vi "Gain compensation.vi"(5 "A":dbl=1.2727, 7 "b":dbl=-0.169, 10 "sampling frequency":dbl=50.0, 11 "Data":dbl[](array[numeric])) -> (3 "compensated":dbl[](array[numeric]))   [LabVIEW 2012]
uses:
  <vilib>/Analysis/2dsp.llb/Real FFT.vi
  <vilib>/Analysis/2dsp.llb/Inverse Real FFT.vi
  <vilib>/Analysis/NI_AALPro.lvlib
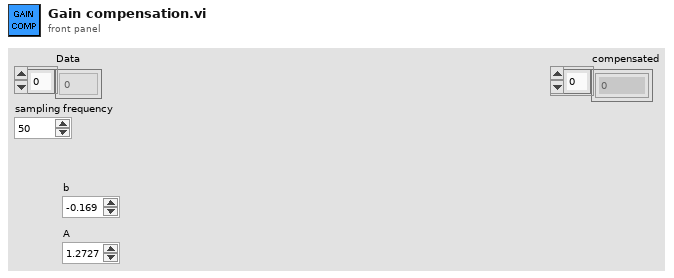
[diagram p1: front panel]
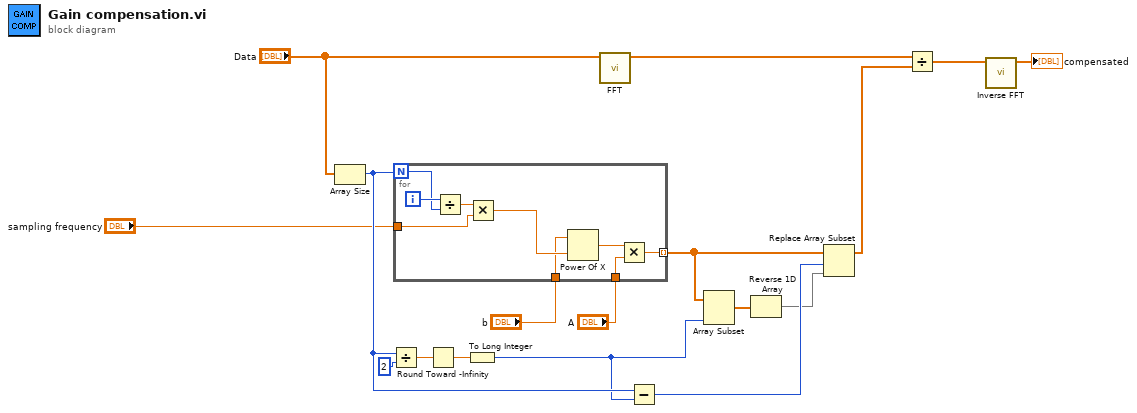
[diagram p0: block diagram]
diagram:
  n1 = Array Size(array="Data") -> (size(s)=w10:i32)
  n2 = Divide(x=w10, y=2) -> (x/y=w14:dbl)
  n3 = for {
    N: w10 -> [w18]
    tunnel: "sampling frequency" -> [w24]
    tunnel: "b" -> [w22]
    tunnel: "A" -> [w20]
    tunnel: [w19] -> w11 mode=indexing
    i -> [w26]
    n4 = Divide(x=w26, y=w18) -> (x/y=w25:dbl)
    n5 = Multiply(x=w25, y=w24) -> (x*y=w23:dbl)
    n6 = Power Of X(1:w23, 2:w22) -> (0:w21:dbl)
    n7 = Multiply(x=w21, y=w20) -> (x*y=w19:dbl)
  }
  n8 = Round Toward -Infinity(1:w14) -> (0:w13:dbl)
  n9 = To Long Integer(number=w13) -> (32bit integer=w9:i32)
  n10 = call-poly <vilib>:"FFT.vi"("X"="Data") -> ("FFT {X}"=w6:cdb[])  [unwired: 9 in, 1 out]
  n11 = Subtract(x=w10, y=w9) -> (x-y=w8:i32)
  n12 = Array Subset(array=w11, length=w9) -> (w12:dbl[])  [unwired: 1 in]
  n13 = Reverse 1D Array(array=w12) -> (reversed array=w7:dbl[])
  n14 = Replace Array Subset(array=w11, new element=w7, index=w8) -> (w5:dbl[])
  n15 = Divide(x=w6, y=w5) -> (x/y=w4:cdb[])
  n16 = call-poly <vilib>:"Inverse FFT.vi"("FFT {X}"=w4) -> ("X"=→"compensated":dbl[])  [unwired: 9 in, 1 out]
